vi "GetLibraryExists.vi"(8 "ErrorIn":errorcluster caption="Error In(no Error)", 9 "LibraryName":string, 11 "ReferenceIn":refnum<class "ErrorDefinitionSQLite.lvclass"> caption="Reference In") -> (0 "ErrorOut":errorcluster caption="Error Out", 1 "Exists":bool, 2 "NewNeeded":bool, 3 "ReferenceOut":refnum<class "ErrorDefinitionSQLite.lvclass"> caption="Reference Out", 4 "Full":bool)   [LabVIEW 2021, in "ErrorDefinitionSQLite.lvclass"]
uses:
  ErrorDefinitionSQLite.lvclass
  <vilib>/drjdpowell/SQLite Library/SQL Connection/Execute SQL.vi
  <vilib>/drjdpowell/SQLite Library/SQLite.lvlib
  <vilib>/drjdpowell/SQLite Library/SQL Connection/Connection.lvclass
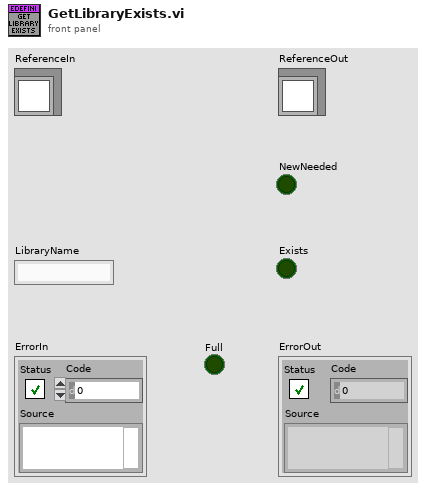
[diagram p1: front panel]
types:
  T1 = typedef "ErrorDefinitionSQLite.lvclass/ObjectAttributes.ctl" = cluster{"Path":path, "SQLiteRef":refnum<class "Connection.lvclass">, "EndOfRange":i32, "DefaultLibrarySize":i32, "StartOfRange":i32}
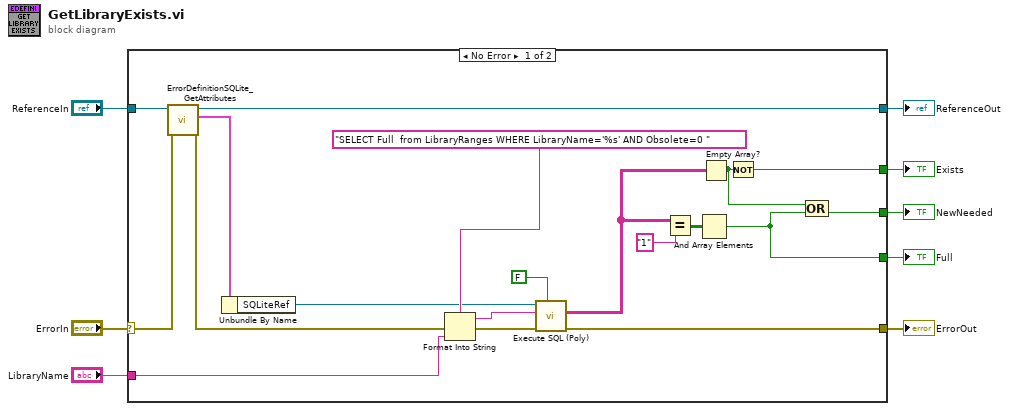
[diagram p0: block diagram]
diagram:
  n1 = case shown="No Error" "ErrorIn" {
    selector: "ErrorIn" -> [w27 w29]
    tunnel: [w24 w29] -> w7
    tunnel: [w22 w28] -> w5
    tunnel: "ReferenceIn" -> [w23 w28]
    tunnel: "LibraryName" -> [w17 _]
    tunnel: [w11 _] -> w3
    tunnel: [w15 _] -> w2
    tunnel: [w9 _] -> w1
    frame No Error {
      n2 = call "ErrorDefinitionSQLite_GetAttributes.vi"("ErrorIn"=w27, "Reference in"=w23) -> ("ErrorOut"=w25:errorcluster, "Data"=w21:T1, "Reference out"=w22:refnum<class "ErrorDefinitionSQLite.lvclass">)  [unwired: 6 in, 1 out]
      n3 = Unbundle By Name(w21) -> ("SQLiteRef"=w16:refnum<class "Connection.lvclass">)
      n4 = Format Into String(format string="SELECT Full  from LibraryRanges WHERE LibraryName='%s' AND Obsolete=0 " ("SQL"), error in=w25, w17) -> (resulting string=w18:string, error out=w26:errorcluster)  [unwired: 1 in]
      n5 = call-poly <vilib>:"Execute SQL (Poly).vi"("Use SAVEPOINT"=FALSE, "error in (no error)"=w26, "SQL"=w18, "SQLite Connection in"=w16) -> ("error out"=w24:errorcluster, "Result Set"=w14:string[][])  [unwired: 4 in, 2 out]
      n6 = Equal?(x=w14, y="1") -> (x = y?=w12:bool[][])
      n7 = And Array Elements(Boolean array=w12) -> (logical AND=w9:bool)
      n8 = Empty Array?(array=w14) -> (empty?=w10:bool)
      n9 = Not(x=w10) -> (.not. x?=w15:bool)
      n10 = Compound Arithmetic op=OR(w10, w9) -> (w11:bool)
    }
    frame Error {
    }
  }
  "ErrorOut" <- w7
  "ReferenceOut" <- w5
  "NewNeeded" <- w3
  "Exists" <- w2
  "Full" <- w1
